vi "Self-Test.vi"(8 "error in (no error)":errorcluster, 11 "Instrument in":refnum<class "Instrument.lvclass">) -> (0 "error out":errorcluster, 1 "Self-Test Result Message":string, 2 "Self-Test Result Code":i32, 3 "Instrument out":refnum<class "Instrument.lvclass">)   [LabVIEW 2017, in "Instrument.lvlib" / "Instrument.lvclass"]
doc: "Runs an Instruments internal Self-Test procedure and returns a Self-Test code and message. An empty string and return code of 0 represents a successful self-test. If the internal self-test throws an error it will, in general, return the error as a self-test code and string rather than on the error wire."
uses:
  Instrument.lvclass
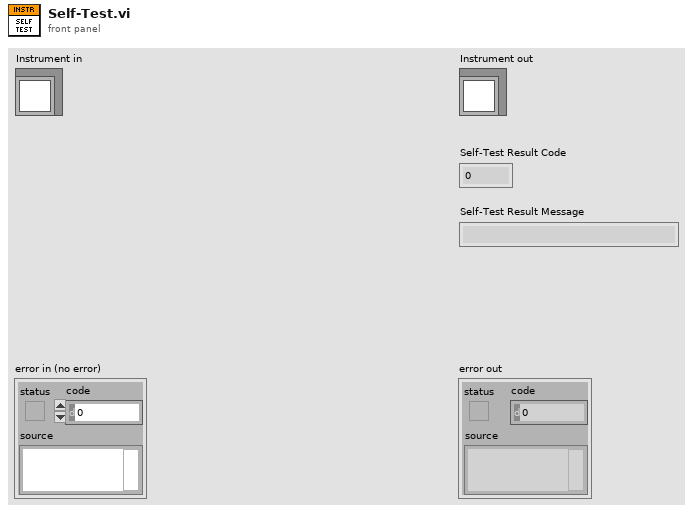
[diagram p1: front panel]
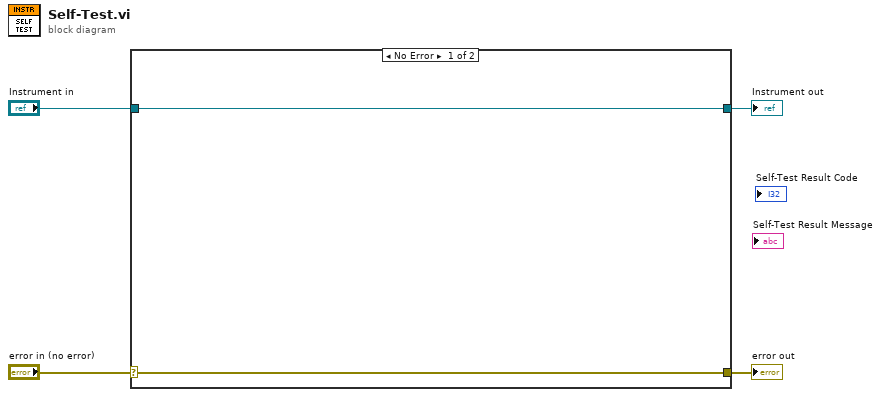
[diagram p0: block diagram]
diagram:
  n1 = case shown="No Error" "error in (no error)" {
    selector: "error in (no error)" -> [w5 w8]
    tunnel: [w5 w8] -> w3
    tunnel: [w6 w7] -> w1
    tunnel: "Instrument in" -> [w6 w7]
    frame No Error {
    }
    frame Error {
    }
  }
  "error out" <- w3
  "Instrument out" <- w1
